vi "Ultrasonic_Open.vi"(2 "error in (no error)":errorcluster, 3 "DIO Channel":T4, 4 "Scaling factor (s/in)":dbl) -> (0 "error out":errorcluster, 1 "SonarMB1010DigitalDevRef":T1={"CounterDevRef"={"DevStatus"={"status"=FALSE, "code"=0, "source"=""}, "CntIndex"=enum."Invalid"}, "Scaling factor (s/in)"=0.000147})   [LabVIEW 2016, in "ArgosLib.lvlib"]
uses:
  <vilib>/Rock Robotics/SystemInterfaces/DIO/FPGA_DIOChannel.ctl
  <vilib>/Rock Robotics/WPI/Ultrasonic/WPI_SonarMB1010DigitalDeviceRef.ctl
  <vilib>/Rock Robotics/WPI/Counter/WPI_CounterDevRef.ctl
  <vilib>/Rock Robotics/SystemInterfaces/Counter/FPGA_CounterCtrSystemIndex.ctl
  <vilib>/Rock Robotics/WPI/Counter/WPI_CounterDigitalInputToDigitalSource.vi
  <vilib>/Rock Robotics/WPI/Counter/WPI_CounterOpen Semi Period Mode.vi
  ArgosLib.lvlib
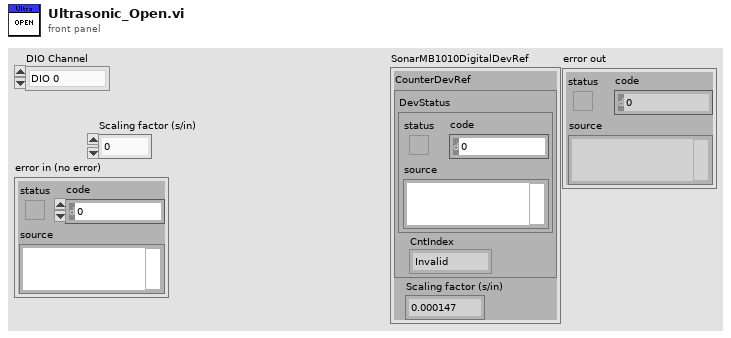
[diagram p1: front panel]
types:
  T1 = typedef "WPI_SonarMB1010DigitalDeviceRef.ctl" = cluster{"CounterDevRef":T2, "Scaling factor (s/in)":dbl}
  T2 = typedef "WPI_CounterDevRef.ctl" = cluster{"DevStatus":errorcluster, "CntIndex":T3}
  T3 = typedef "FPGA_CounterCtrSystemIndex.ctl" = enum8{"Ctr 0", "Ctr 1", "Ctr 2", "Ctr 3", "Ctr 4", "Ctr 5", "Ctr 6", "Ctr 7", "Invalid"}
  T4 = typedef "FPGA_DIOChannel.ctl" = enum8{"DIO 0", "DIO 1", "DIO 2", "DIO 3", "DIO 4", "DIO 5", "DIO 6", "DIO 7", "DIO 8", "DIO 9", "DIO MXP 0", "DIO MXP 1", "DIO MXP 2", "DIO MXP 3", "DIO MXP 4", "DIO MXP 5", "DIO MXP 6", "DIO MXP 7", "DIO MXP 8", "DIO MXP 9", "DIO MXP 10", "DIO MXP 11", "DIO MXP 12", "DIO MXP 13", "DIO MXP 14", "DIO MXP 15", "SPI Port CS1", "SPI Port CS2", "SPI Port CS3", "SPI Port MISO", "SPI Port MOSI", "Invalid"}
  T5 = typedef "WPI_DigitalInputDevRef.ctl" = cluster{"DevStatus":errorcluster, "DIO Channel":T4}
  T6 = typedef "FPGA_CounterEncoderSourceConvertionLVSourceType.ctl" = cluster{"DevStatus":errorcluster, "AnalogTriggerMode?":bool, "DigitalMode":cluster{"DIO Channel":T7}, "AnalogTriggerMode":cluster{"AnalogTriggerIndex":T8, "OutputType":T9}}
  T7 = typedef "FPGA_DIODigitalSourceChannel.ctl" = enum8{"DIO 0", "DIO 1", "DIO 2", "DIO 3", "DIO 4", "DIO 5", "DIO 6", "DIO 7", "DIO 8", "DIO 9", "DIO MXP 0", "DIO MXP 1", "DIO MXP 2", "DIO MXP 3", "DIO MXP 4", "DIO MXP 5", "DIO MXP 6", "DIO MXP 7", "DIO MXP 8", "DIO MXP 9", "DIO MXP 10", "DIO MXP 11", "DIO MXP 12", "DIO MXP 13", "DIO MXP 14", "DIO MXP 15", "Disabled"}
  T8 = typedef "FPGA_AnalogTriggerIndex.ctl" = enum8{"Trig 0", "Trig 1", "Trig 2", "Trig 3", "Trig 4", "Trig 5", "Trig 6", "Trig 7", "Invalid"}
  T9 = typedef "FPGA_AnalogTriggerOutType.ctl" = enum16{"InWindow", "TriggerState", "Rising", "Falling"}
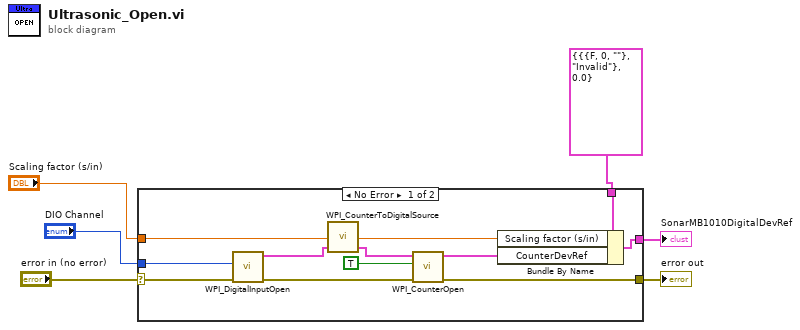
[diagram p0: block diagram]
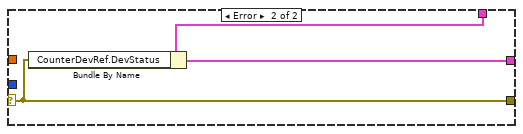
[diagram p2: hidden frame]
diagram:
  n1 = case shown="No Error" "error in (no error)" {
    selector: "error in (no error)" -> [w17 w18]
    tunnel: "DIO Channel" -> [w16 _]
    tunnel: "Scaling factor (s/in)" -> [w11 _]
    tunnel: T1 {"CounterDevRef"={"DevStatus"={"status"=FALSE, "code"=0, "source"=""}, "CntIndex"=enum."Invalid"}, "Scaling factor (s/in)"=0.0} ("SonarMB1010DigitalDevRef") -> [w9 w20]
    tunnel: [w8 w19] -> w2
    tunnel: [w7 w18] -> w1
    frame No Error {
      n2 = call <vilib>:"WPI_DigitalInputOpen.vi"("error in (no error)"=w17, "DIO Channel"=w16) -> ("error out"=w12:errorcluster, "DigitalInputDevRef"=w14:T5)  [unwired: 8 in]
      n3 = call-poly <vilib>:"WPI_CounterToDigitalSource.vi"("DigitalInputDevRef"=w14) -> ("Digital Source"=w15:T6)  [unwired: 6 out]
      n4 = call-poly <vilib>:"WPI_CounterOpen.vi"("error in (no error)"=w12, "High Pulse (T)"=TRUE, "Source"=w15) -> ("error out"=w7:errorcluster, "CounterDevRef"=w10:T2)  [unwired: 2 in, 5 out]
      n5 = Bundle By Name(cluster=w9, "Scaling factor (s/in)"=w11, "CounterDevRef"=w10) -> (w8:T1)
    }
    frame Error {
      n6 = Bundle By Name(cluster=w20, "CounterDevRef.DevStatus"=w18) -> (w19:T1)
    }
  }
  "SonarMB1010DigitalDevRef" <- w2
  "error out" <- w1
